vi "class_data.vi"() -> ()   [LabVIEW 2010, in "LightSourceMH110124MaiTai.lvclass"]
uses:
  LightSourceMH110124MaiTai.lvclass
panel:
  out "wavelength maximum":dbl[unit]
  out "wavelength minimum":dbl[unit]
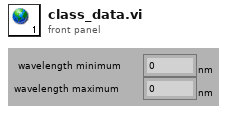
[diagram p1: front panel]
diagram:
